vi "Open Connection.vi"(4 "error in (no error)":errorcluster, 5 "Password (\"\")":string, 6 "Username (\"\")":string, 7 "ODBC DB Name (\"\")":string) -> (0 "error out":errorcluster, 3 "Connection Refnum":T1)   [LabVIEW 2011]
doc: "Réalise l'ensemble des étapes nécéssaires à la mise en place de la connection avec la base de données. Etablit le cas échéant l'utilisation des transactions."
uses:
  SQL Controls/Connection Refnum.ctl
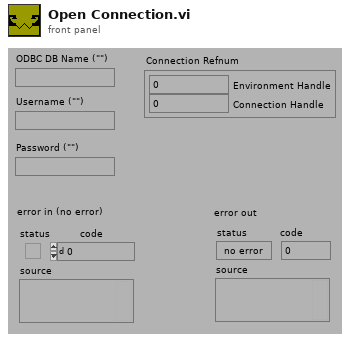
[diagram p1: front panel]
types:
  T1 = typedef "Connection Refnum.ctl" = cluster{"Environment Handle":i32, "Connection Handle":i32}
  T2 = cluster{"Environment Handle":i32, "Connection Handle":i32}
  T3 = enum16{"NOPE", "SQL_HANDLE_ENV", "SQL_HANDLE_DBC", "SQL_HANDLE_STMT", "SQL_HANDLE_DESC"}
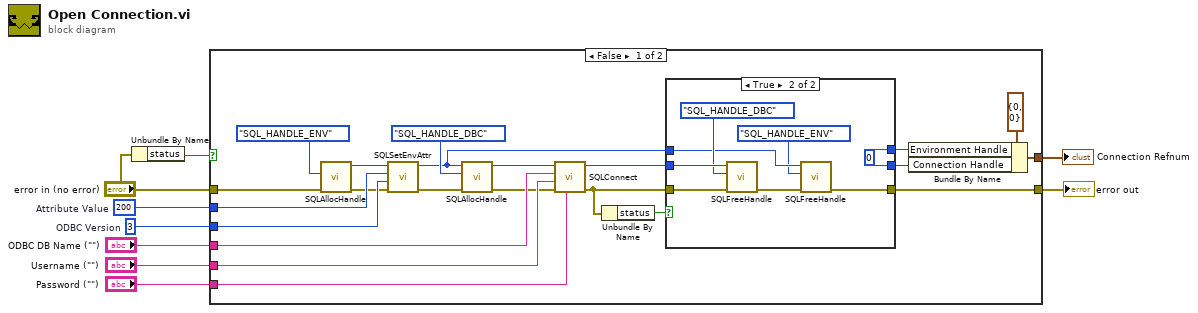
[diagram p0: block diagram]
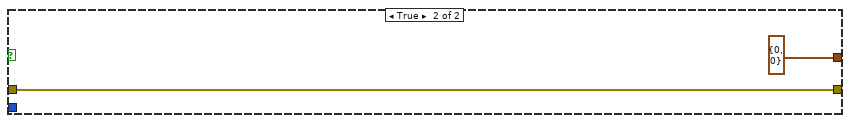
[diagram p3: hidden frame]
diagram:
  w5 = u32 3  # ODBC Version
  w6 = 200  # Attribute Value
  n1 = Unbundle By Name("error in (no error)") -> ("status"=w1:bool)
  n2 = case shown="False" w1 {
    tunnel: "Username (\"\")" -> [w31 _]
    tunnel: "ODBC DB Name (\"\")" -> [w30 _]
    tunnel: "Password (\"\")" -> [w29 _]
    tunnel: w6 -> [w25 _]
    tunnel: w5 -> [w24 _]
    tunnel: [w19 T2 {"Environment Handle"=0, "Connection Handle"=0} ("Connection Refnum")] -> w4
    tunnel: [w11 w44] -> w3
    tunnel: "error in (no error)" -> [w10 w44]
    frame False {
      n3 = call "SQLAllocHandle.vi"("error in (no error)"=w10, "HandleType"=T3."SQL_HANDLE_ENV") -> ("error out"=w16:errorcluster, "OutputHandle"=w21:i32)  [unwired: 1 in, 3 out]
      n4 = call "SQLSetEnvAttr.vi"("error in (no error)"=w16, "AttributeValue"=w24, "AttributePosition"=w25, "InputHandle"=w21) -> ("error out"=w15:errorcluster, "OutputHandle"=w26:i32)  [unwired: 2 out]
      n5 = call "SQLAllocHandle.vi"("error in (no error)"=w15, "HandleType"=T3."SQL_HANDLE_DBC", "InputHandle"=w26) -> ("error out"=w14:errorcluster, "OutputHandle"=w23:i32)  [unwired: 3 out]
      n6 = call "SQLConnect.vi"("Password"=w29, "error in (no error)"=w14, "UserName"=w31, "ServerName"=w30, "InputHandle"=w23) -> ("error out"=w12:errorcluster, "OutputHandle"=w22:i32)  [unwired: 2 out]
      n7 = Unbundle By Name(w12) -> ("status"=w13:bool)
      n8 = case shown="True" w13 {
        tunnel: w22 -> [w33 w42]
        tunnel: w26 -> [w34 w37]
        tunnel: [w34 w41] -> w18
        tunnel: [w33 w41] -> w17
        tunnel: [w32 w35] -> w11
        tunnel: w12 -> [w32 w40]
        frame False {
        }
        frame True {
          w41 = 0 ("OutputHandle")
          n9 = call "SQLFreeHandle.vi"("error in (no error)"=w40, "HandleType"=T3."SQL_HANDLE_DBC", "InputHandle"=w42) -> ("error out"=w38:errorcluster)  [unwired: 4 out]
          n10 = call "SQLFreeHandle.vi"("error in (no error)"=w38, "HandleType"=T3."SQL_HANDLE_ENV", "InputHandle"=w37) -> ("error out"=w35:errorcluster)  [unwired: 4 out]
        }
      }
      n11 = Bundle By Name(cluster=T2 {"Environment Handle"=0, "Connection Handle"=0} ("Connection Refnum"), "Environment Handle"=w18, "Connection Handle"=w17) -> (w19:T2)
    }
    frame True {
    }
  }
  "Connection Refnum" <- w4
  "error out" <- w3
